vi "Launch SCH Protection RT.vi"() -> ()   [LabVIEW 2018]
doc: "Author: Scott Hannahs <sth@magnet.fsu.edu>\nCopyright 2018 Florida State University, All rights reserved."
panel:
  out "error out":errorcluster
  in  "VI Name":string="SCH Protection-RT Host.vi"
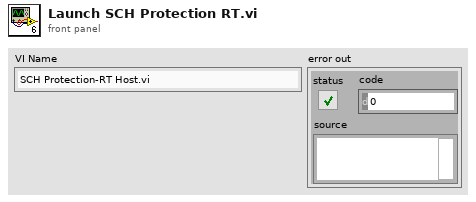
[diagram p1: front panel]
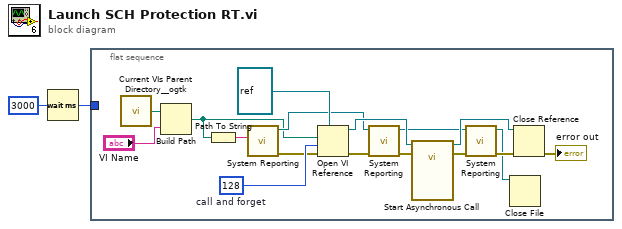
[diagram p0: block diagram]
diagram:
  n1 = Wait (ms)(milliseconds to wait=u32 3000) -> (millisecond timer value=w1:u32)
  n2 = flat-sequence {
    tunnel: w1 -> [_]
    frame #0 {
      w19 = 128  # call and forget
      n3 = call <userlib>:"Current VIs Parent Directory__ogtk.vi"() -> ("Parent Directory (+ Relative)"=w6:path)  [unwired: 5 in]
      n4 = Build Path(base path=w6, name or relative path="VI Name") -> (appended path=w4:path)
      n5 = Path To String(path=w4) -> (string=w3:string)
      n6 = call "System Reporting.vi"("String"=w3) -> ("Error Out"=w8:errorcluster, "Byte Stream File out"=w13:refnum<file>)  [unwired: 9 in]
      n7 = Open VI Reference(type specifier VI Refnum (for type only)=refnum<vi> refnum, vi path=w4, options=w19, error in (no error)=w8) -> (vi reference=w17:refnum<vi>, error out=w14:errorcluster)  [unwired: 2 in]
      n8 = call "System Reporting.vi"("Error In"=w14, "Byte Stream File in"=w13) -> ("Error Out"=w11:errorcluster, "Byte Stream File out"=w12:refnum<file>)  [unwired: 8 in]
      n9 = call-by-ref "Start Asynchronous Call"(reference=w17, error in=w11) -> (reference out=w16:refnum<vi>, error out=w10:errorcluster)  [unwired: 12 in]
      n10 = call "System Reporting.vi"("Error In"=w10, "Byte Stream File in"=w12) -> ("Error Out"=w9:errorcluster, "Byte Stream File out"=w7:refnum<file>)  [unwired: 8 in]
      n11 = Close File(refnum=w7) -> ()  [unwired: 1 in, 2 out]
      n12 = Close Reference(reference=w16, error in (no error)=w9) -> (error out=→"error out":errorcluster)
    }
  }
